vi "Multiple Record Fetch (Host).vi"() -> ()   [LabVIEW 2021]
doc: "Use this VI as a template to design an application that acquires multiple records of data from the NI PXIe-5170R/5171R."
uses:
  <instrlib>/_niInstr/Multirecord Acquisition/Interface/v1/Host/Public/Requested Record Info.ctl
  <instrlib>/_niInstr/Multirecord Acquisition/Interface/v1/Host/Public/Fetch Relative To Enum.ctl
  <instrlib>/_niInstr/Multirecord Acquisition/Interface/v1/Host/Public/Full Record Status.ctl
  <instrlib>/_niInstr/Multirecord Acquisition/Interface/v1/Host/Public/Record State.ctl
  <instrlib>/_niInstr/Multirecord Acquisition/Interface/v1/Host/Public/Record Status.ctl
  <instrlib>/HSAI-RIO/Types/v1/Host/Typedefs/Temp Source.ctl
  <instrlib>/_niInstr/Data Trigger/v1/Shared/Public/Level Configuration Trigger When.ctl
  <vilib>/FPGAPlugInAG/PXIe-5170R (8CH)/niLvFpga_Open_PXIe-5170R (8CH).vi
  <vilib>/rvi/interface/common/dynamic/niFpgaDynamicAddResources.vi
  <vilib>/FPGAPlugInAG/Dynamic/niLvFpga_Close_Dynamic.vi
  <vilib>/rvi/interface/nirviOpenFPGA/nirviOpenFPGA.xnode
  FPGA Bitfiles/Multirecord_Acquisition_NI_PXIe-5170R_8CH.lvbitx
  <vilib>/rvi/interface/nirviCloseFPGA/nirviCloseFPGA.xnode
  Device Session/Device Session.lvclass
  <instrlib>/HSAI-RIO/Types/v1/Host/niHSAI Types v1 Host.lvlib
  <instrlib>/_niInstr/Data Trigger/v1/Shared/niInstr Data Trigger v1 Shared.lvlib
  <instrlib>/_niInstr/Multirecord Acquisition/Interface/v1/Host/niInstr Multirecord Acquisition v1 Host.lvclass
panel:
  out "Record Number displayed":u64=15
  in  "Fetch?":bool
  out "current record status":T1={"started"=TRUE, "reference trigger detected"=FALSE, "reference trigger sample number"=0, "samples written"=62127289728}
  out "overflow occurred":bool
  out "records done":u64=16
  out "record status":T2={"state"=enum."Completed", "ref trigger detected"=TRUE, "ref trigger sample number"=1021, "first pretrigger sample number"=21, "samples written"=100021, "current read position"=100021, "first valid sample"=0, "last valid sample to request"=100020, "timestamps"=[0]}
  out "done":bool
  out "number of outstanding record requests":u32
  in  "pretrigger samples":u64=1000
  out "Loop count":i32=1905
  out "fetch backlog":u64
  in  "fetch offset":i64
  in  "fetch relative to":T4=enum."First Pretrigger Sample"
  in  "record number":u64=15
  in  "onboard sample clock rate":dbl(ring)=250000000.0 items=["250 MHz"=250000000.0, "200 MHz"=200000000.0, "150 MHz"=150000000.0]
  out "Waveform Graph":T5(graph)
  out "fpga temperature (°C)":dbl(slide)=45.279516601562534 scale=0.0..96.0 scale format="%#_6p"
  out "power consumption (W)":dbl(slide)=20.759999999999998 scale=0.0..38.25 scale format="%#_6p"
  out "number of records fetched":u64=1906
  in  "display":bool
  in  "stop":bool
  in  "number of samples":u64=10000
  in  "number of records":u64=1
  in  "channels to configure":string="0"
  out "error out":errorcluster
  out "requested records info":T6[](array[typedef])=[{"number of samples"=100000, "starting sample number"=21, "number of channels"=1, "timestamps"=[0]}]
  in  "RIO Device":tag="5170"
  # "RIO Device"
  # "Channels"
  # "Acquisition Settings"
  # "Records Fetched Info"
  # "System Monitor"
  # "Clocking"
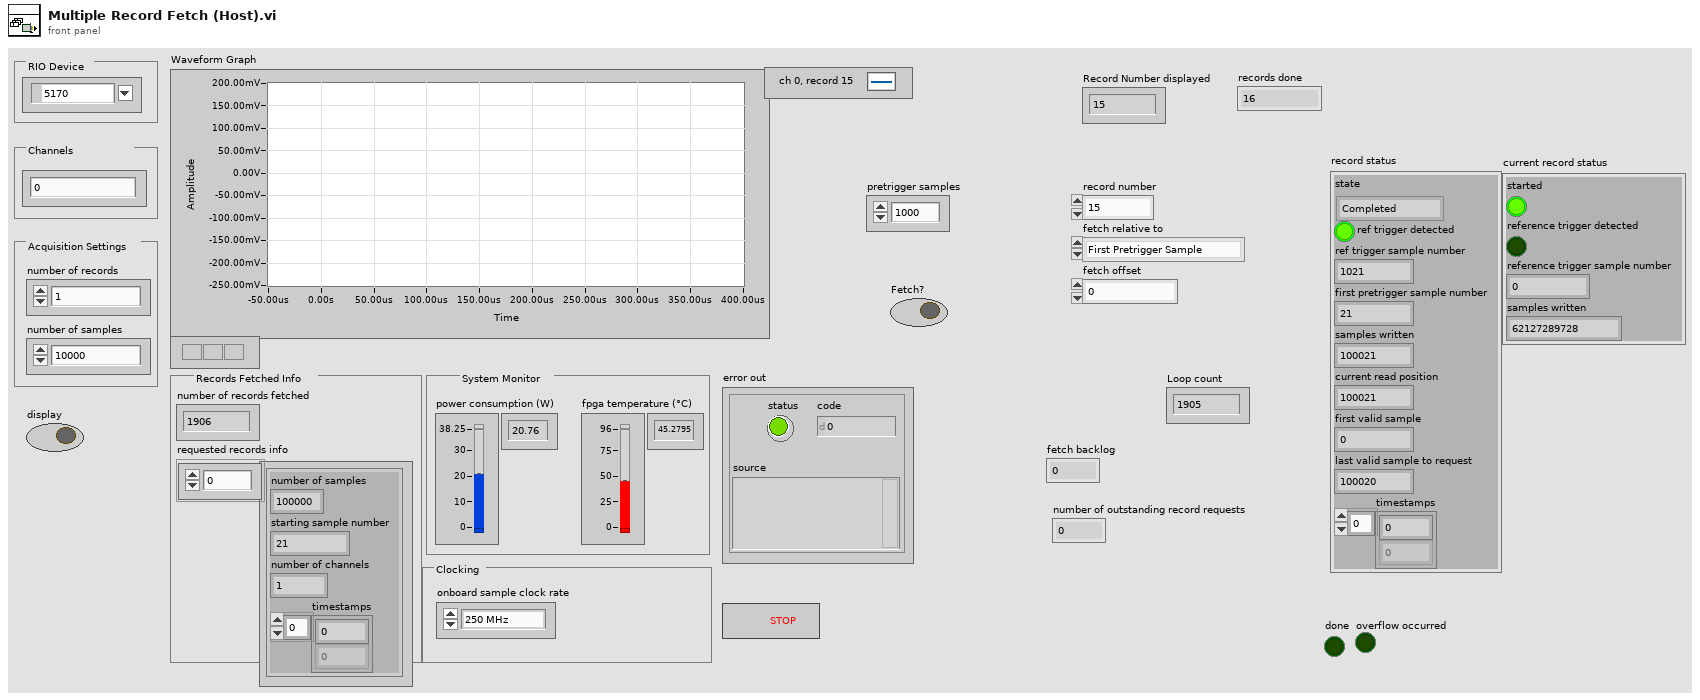
[diagram p1: front panel]
types:
  T1 = typedef "niInstr Multirecord Acquisition v1 Host.lvclass/Record Status.ctl" = cluster{"started":bool, "reference trigger detected":bool, "reference trigger sample number":u64, "samples written":u64}
  T2 = typedef "niInstr Multirecord Acquisition v1 Host.lvclass/Full Record Status.ctl" = cluster{"state":T3, "ref trigger detected":bool, "ref trigger sample number":u64, "first pretrigger sample number":u64, "samples written":u64, "current read position":u64, "first valid sample":u64, "last valid sample to request":u64, "timestamps":u64[]}
  T3 = typedef "niInstr Multirecord Acquisition v1 Host.lvclass/Record State.ctl" = enum16{"Not Started", "Being Acquired", "Completed", "Overwritten"}
  T4 = typedef "niInstr Multirecord Acquisition v1 Host.lvclass/Fetch Relative To Enum.ctl" = enum16{"First Sample", "Reference Trigger Sample", "First Pretrigger Sample", "Most Recent Sample", "Current Read Position"}
  T5 = cluster{"relativeX":dbl, "sample rate":dbl, "data in":dbl[]}[]
  T6 = typedef "niInstr Multirecord Acquisition v1 Host.lvclass/Requested Record Info.ctl" = cluster{"number of samples":u64, "starting sample number":u64, "number of channels":u64, "timestamps":u64[]}
  T7 = typedef "niInstr Data Trigger v1 Shared.lvlib/Level Configuration Trigger When.ctl" = enum8{"Trigger Above", "Trigger Below"}
  T8 = enum16{"Immediate", "A", "B", "OR", "AND", "A THEN B", "B THEN A", "High Resolution"}
  T9 = typedef "niHSAI Types v1 Host.lvlib/Temp Source.ctl" = enum8{"Device Temperature", "Thermal Shutdown Margin", "FPGA Temperature", "FPGA Temperature Limit"}
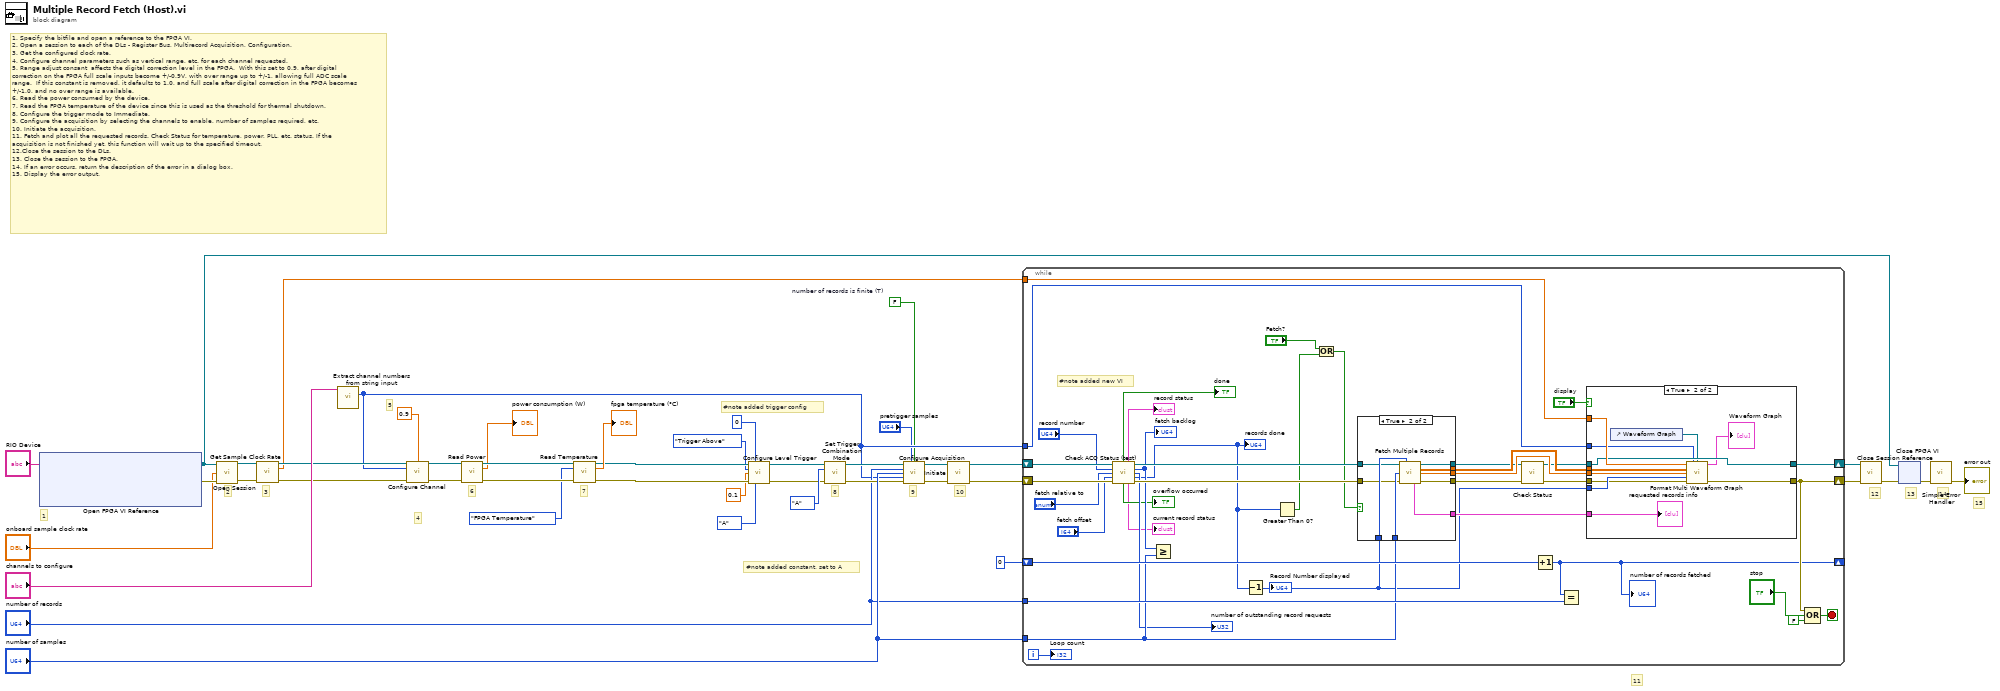
[diagram p0: block diagram]
diagram:
  w1 = FALSE  # number of records is finite (T)
  # "#note added constant, set to A"
  # "#note added trigger config"
  # "5"
  # "7"
  # "6"
  # "8"
  # "15"
  # "14"
  # "13"
  # "12"
  # "11"
  # "10"
  # "9"
  # "4"
  # "3"
  # "1"
  # "2"
  # "1. Specify the bitfile and open a reference to the FPGA VI.\n2. Open a session to each of the DLs - Register Bus, Multirecord Acquisition, Configuration.\n3. Get the configured clock rate.\n4. Configure channel parameters such as vertical range, etc. for each channel requested.\n5. Range adjust consant  affects the digital correction level in the FPGA.  With this set to 0.9, after digital correction on the FPGA full scale inputs become +/-0.9V, with over range up to +/-1, allowing full ADC scale range.  If this constant is removed, it defaults to 1.0, and full scale after digital correction in the FPGA becomes +/-1.0, and no over range is available.\n6. Read the power consumed by the device.\n7. Read the FPGA temperature of the device since this is used as the threshold for thermal shutdown.\n8. Configure the trigger mode to Immediate.\n9. Configure the acquisition by selecting the channels to enable, number of samples required, etc.\n10. Initiate the acquisition.\n11. Fetch and plot all the requested records. Check Status for temperature, power, PLL, etc. status. If the acquisition is not finished yet, this function will wait up to the specified timeout.\n12.Close the session to the DLs.\n13. Close the session to the FPGA.\n14. If an error occurs, return the description of the error in a dialog box.\n15. Display the error output."
  n1 = xnode "Open FPGA VI Reference"("resource name"="RIO Device") -> ("FPGA VI Reference Out"=w29:refnum<k20>, "error out"=w30:errorcluster)  [unwired: 1 in]
  n2 = call "Open Session.vi"("fpga reference in"=w29, "adc clock rate (Hz)"="onboard sample clock rate", "error in"=w30) -> ("device session out"=w34:refnum<class "Device Session.lvclass">, "error out"=w35:errorcluster)  [unwired: 11 in]
  n3 = call "Get Sample Clock Rate.vi"("device session in"=w34, "error in"=w35) -> ("device session out"=w33:refnum<class "Device Session.lvclass">, "sample clock rate (Hz)"=w15:dbl, "error out"=w32:errorcluster)  [unwired: 11 in]
  n4 = call "Extract channel numbers from string input.vi"("channel input"="channels to configure") -> ("array of chans"=w12:u32[])  [unwired: 13 in, 1 out]
  n5 = call "Configure Channel.vi"("device session in"=w33, "range adjust"=0.9, "channels"=w12, "error in"=w32) -> ("device session out"=w20:refnum<class "Device Session.lvclass">, "error out"=w19:errorcluster)  [unwired: 10 in]
  n6 = call "Read Power.vi"("device session in"=w20, "error in"=w19) -> ("device session out"=w24:refnum<class "Device Session.lvclass">, "power (W)"=→"power consumption (W)":dbl, "error out"=w23:errorcluster)  [unwired: 11 in]
  n7 = call "Read Temperature.vi"("device session in"=w24, "source"=Temp_Source."FPGA Temperature", "error in"=w23) -> ("device session out"=w10:refnum<class "Device Session.lvclass">, "temperature (°C)"=→"fpga temperature (°C)":dbl, "error out"=w9:errorcluster)  [unwired: 10 in]
  n8 = call "Configure Level Trigger.vi"("device session in"=w10, "trigger source"=u8 0, "trigger when"=Level_Configuration_Trigger_When."Trigger Above", "trigger level (V)"=0.1, "error in"=w9, "instance"=enum16{"A", "B"}."A") -> ("device session out"=w8:refnum<class "Device Session.lvclass">, "error out"=w7:errorcluster)  [unwired: 8 in]
  n9 = call "Set Trigger Combination Mode.vi"("device session in"=w8, "mode"=T8."A", "error in"=w7) -> ("device session out"=w26:refnum<class "Device Session.lvclass">, "error out"=w25:errorcluster)  [unwired: 11 in]
  n10 = call "Configure Acquisition.vi"("device session in"=w26, "pretrigger samples"="pretrigger samples", "number of records is finite (T)"=w1, "number of records"="number of records", "number of samples"="number of samples", "channels to store"=w12, "error in"=w25) -> ("device session out"=w44:refnum<class "Device Session.lvclass">, "error out"=w43:errorcluster)  [unwired: 6 in, 1 out]
  n11 = call "Initiate.vi"("device session in"=w44, "error in"=w43) -> ("device session out"=w41:refnum<class "Device Session.lvclass">, "error out"=w42:errorcluster)  [unwired: 12 in]
  n12 = while {
    tunnel: "number of samples" -> [w56]
    tunnel: w15 -> [w81]
    shift-right: [w67] -> w36
    shift-left: w42 -> [w63]
    shift-right: [w77] -> w37
    shift-left: w41 -> [w65]
    tunnel: w12 -> [w76]
    shift-right: [w66] -> _
    shift-left: u64 0 -> [w69]
    tunnel: "number of records" -> [w68]
    i -> [w61]
    stop <- w70 stop-if-true
    # "#note added new VI"
    n13 = call "Check ACQ Status (test).vi"("device session in"=w65, "record number"="record number", "fetch relative to"="fetch relative to", "fetch offset"="fetch offset", "error in"=w63) -> ("done"=→"done":bool, "record status"=→"record status":T2, "device session out"=w64:refnum<class "Device Session.lvclass">, "fetch backlog"=w57:u64, "number of outstanding record requests"=→"number of outstanding record requests":u32, "records done"=w47:u64, "overflow occurred"=→"overflow occurred":bool, "current record status"=→"current record status":T1, "error out"=w62:errorcluster)  [unwired: 2 in]
    "fetch backlog" <- w57
    "records done" <- w47
    n14 = Greater Or Equal?(x=w57, y=w56) -> ()  [unwired: 1 out]
    n15 = Decrement(x=w47) -> (x-1=w45:u64)
    "Record Number displayed" <- w45
    n16 = Greater Than 0?(x=w47) -> (x > 0?=w46:bool)
    n17 = Or(x="Fetch?", y=w46) -> (x .or. y?=w48:bool)
    n18 = case shown="True" w48 {
      tunnel: [_ w93] -> w82
      tunnel: [_ w92] -> w79
      tunnel: [_ w91] -> w75
      tunnel: [w84 w90] -> w74
      tunnel: [w83 w89] -> w71
      tunnel: w45 -> [_ w88]
      tunnel: w56 -> [_ w87]
      tunnel: w64 -> [w83 w86]
      tunnel: w62 -> [w84 w85]
      frame False {
      }
      frame True {
        n19 = call "Fetch Multiple Records.vi"("device session in"=w86, "starting record"=w88, "number of samples"=w87, "error in"=w85) -> ("device session out"=w89:refnum<class "Device Session.lvclass">, "data"=w93:dbl[][], "relativeX (samples)"=w91:dbl[], "requested records info"=w92:T6[], "error out"=w90:errorcluster)  [unwired: 7 in]
      }
    }
    n20 = call "Check Status.vi"("device session in"=w71, "error in"=w74) -> ("device session out"=w72:refnum<class "Device Session.lvclass">, "error out"=w73:errorcluster)  [unwired: 12 in]
    n21 = Increment(x=w69) -> (x+1=w66:u64)
    "number of records fetched" <- w66
    n22 = Equal?(x=w66, y=w68) -> ()  [unwired: 1 out]
    n23 = case shown="True" "display" {
      tunnel: w82 -> [_ w106]
      tunnel: w81 -> [_ w105]
      tunnel: w79 -> [_ w104]
      tunnel: w73 -> [w95 w100]
      tunnel: [w95 w99] -> w67
      tunnel: w72 -> [w94 w103]
      tunnel: [w94 w103] -> w77
      tunnel: w76 -> [_ w98]
      tunnel: w45 -> [_ w101]
      tunnel: w75 -> [_ w102]
      frame False {
      }
      frame True {
        n24 = control-ref of="Waveform Graph"() -> (w97:refnum<vi>)
        n25 = call "Format Multi Waveform Graph.vi"("sample rate (Hz)"=w105, "array of chans"=w98, "waveform graph"=w97, "data in"=w106, "relativeX (samples)"=w102, "start record number"=w101, "error in"=w100) -> ("waveform out"=→"Waveform Graph":T5, "error out"=w99:errorcluster)  [unwired: 7 in]
        "requested records info" <- w104
      }
    }
    n26 = Compound Arithmetic op=OR(w67, "stop", FALSE ("value")) -> (w70:bool)
    "Loop count" <- w61
  }
  n27 = call "Close Session.vi"("device session in"=w37, "error in"=w36) -> ("error out"=w28:errorcluster)  [unwired: 13 in]
  n28 = xnode "Close FPGA VI Reference"("FPGA VI Reference In"=w29, "error in"=w28) -> ("error out"=w27:errorcluster)
  n29 = call <vilib>:"Simple Error Handler.vi"("error in (no error)"=w27) -> ("error out"=→"error out":errorcluster)  [unwired: 4 in, 4 out]
